vi "ukol2.vi"(2 "Array 2":dbl[][](array[numeric]), 11 "polynomial order":i32=2) -> ()   [LabVIEW 2023]
uses:
  <vilib>/Analysis/6fits.llb/Curve Fitting Criteria.ctl
  <vilib>/Analysis/NI_AALPro.lvlib
panel:
  out "XY Graph":cluster{"Array 2":dbl[], "Array 2":dbl[]}[](graph)
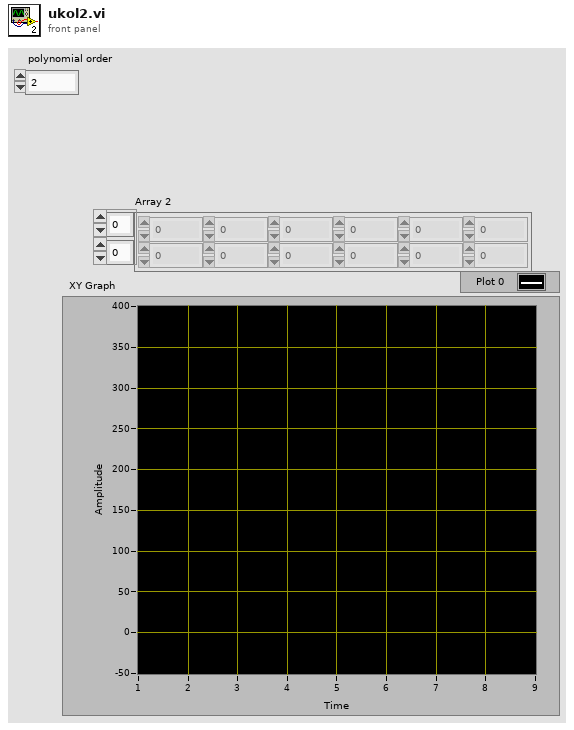
[diagram p1: front panel]
types:
  T1 = typedef "NI_AALPro.lvlib/Curve Fitting Criteria.ctl" = u16
  T2 = cluster{"Array 2":dbl[], "Best Linear Fit":dbl[]}
  T3 = cluster{"Array 2":dbl[], "Best Polynomial Fit":dbl[]}
  T4 = cluster{"Array 2":dbl[], "Best Exponential Fit":dbl[]}
  T5 = cluster{"Array 2":dbl[], "Best Exponential Fit":dbl[]}[]
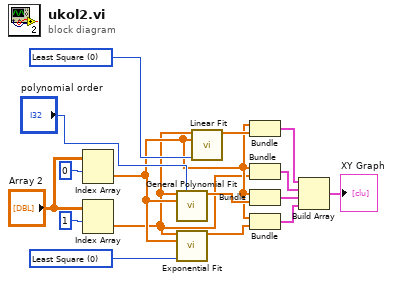
[diagram p0: block diagram]
diagram:
  w7 = T1 0 items=["Least Square", "Least Absolute Residual", "Bisquare"] ("method")
  w13 = T1 0 items=["Least Square", "Least Absolute Residual", "Bisquare"] ("method")
  n1 = Index Array(array="Array 2", index (row)=0) -> (element=w2:dbl[])  [unwired: 1 in]
  n2 = Index Array(array="Array 2", index (row)=1) -> (element=w1:dbl[])  [unwired: 1 in]
  n3 = call <vilib>:"General Polynomial Fit.vi"("Y"=w1, "polynomial order"="polynomial order", "X"=w2) -> ("Best Polynomial Fit"=w4:dbl[])  [unwired: 9 in, 3 out]
  n4 = call <vilib>:"Exponential Fit.vi"("Y"=w1, "X"=w2, "method"=w7) -> ("Best Exponential Fit"=w3:dbl[])  [unwired: 7 in, 5 out]
  n5 = call <vilib>:"Linear Fit.vi"("Y"=w1, "X"=w2, "method"=w13) -> ("Best Linear Fit"=w12:dbl[])  [unwired: 8 in, 4 out]
  n6 = Bundle("Array 2"=w2, "Best Linear Fit"=w12) -> (w11:T2)  [unwired: 1 in]
  n7 = Bundle("Array 2"=w2, "Array 2"=w1) -> (w10:cluster{"Array 2":dbl[], "Array 2":dbl[]})  [unwired: 1 in]
  n8 = Bundle("Array 2"=w2, "Best Polynomial Fit"=w4) -> (w8:T3)  [unwired: 1 in]
  n9 = Bundle("Array 2"=w2, "Best Exponential Fit"=w3) -> (w5:T4)  [unwired: 1 in]
  n10 = Build Array(w11, w10, w8, w5) -> (→"XY Graph":T5)
